vi "Send Set DER Control Msg (Delayed).vi"(7 "Milliseconds To Wait (1000)":i32=1000, 8 "error in":errorcluster, 10 "DER_Control":T1, 11 "SCADA Sub Abstract in":refnum<class "Device Communication and Control Abstract.lvclass">) -> (0 "error out":errorcluster, 3 "dup SCADA Sub Abstract":refnum<class "Device Communication and Control Abstract.lvclass">)   [LabVIEW 2018, in "Device Communication and Control Abstract Actor.lvlib" / "Device Communication and Control Abstract.lvclass"]
uses:
  Device Communication and Control Abstract.lvclass
  C:/Program Files (x86)/National Instruments/LabVIEW 2018/vi.lib/ActorFramework/Actor/Actor.lvclass
  <vilib>/ORNL/CSEISMIC DDS/CSEISMIC DDS Base/Data Types/DER_Control.ctl
  <vilib>/ORNL/CSEISMIC DDS/CSEISMIC DDS Base/Data Types/Controls/DeviceID.ctl
  <vilib>/ActorFramework/Actor/Actor.lvclass/Actor.ctl
  Device Communication and Control Abstract.lvclass/Device Communication and Control Abstract.ctl
  Device Communication and Control Abstract Messages/Set DER Control Msg/Set DER Control Msg.lvclass/Set DER Control Msg.ctl
  Device Communication and Control Abstract Messages/Set DER Control Msg/Set DER Control Msg.lvclass
  C:/Program Files (x86)/National Instruments/LabVIEW 2018/vi.lib/ActorFramework/Message/Message.lvclass
  <vilib>/ActorFramework/Time-Delayed Send Message/Time-Delayed Send Message.vi
  <vilib>/ActorFramework/Actor/Actor.lvclass
  <vilib>/ORNL/CSEISMIC DDS/CSEISMIC DDS Base/CSEISMIC DDS.lvclass
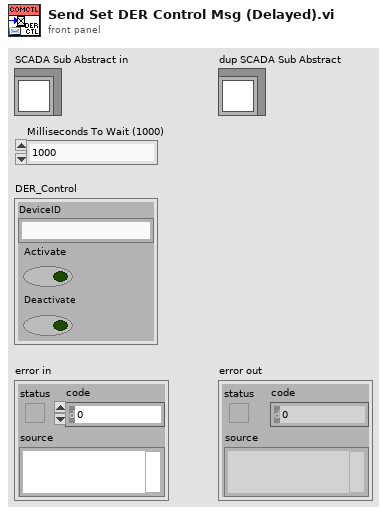
[diagram p1: front panel]
types:
  T1 = typedef "CSEISMIC DDS.lvlib/CSEISMIC DDS.lvclass/DER_Control.ctl" = cluster{"DeviceID":T2, "Activate":bool, "Deactivate":bool}
  T2 = typedef "CSEISMIC DDS.lvlib/CSEISMIC DDS.lvclass/DeviceID.ctl" = string
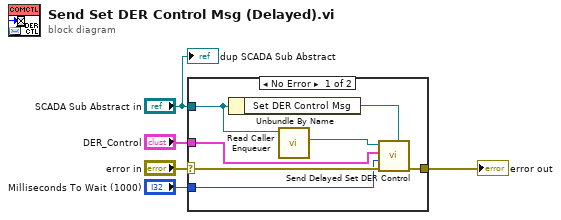
[diagram p0: block diagram]
diagram:
  n1 = case shown="No Error" "error in" {
    selector: "error in" -> [w11 w13]
    tunnel: "SCADA Sub Abstract in" -> [w12 _]
    tunnel: [w10 w13] -> w3
    tunnel: "DER_Control" -> [w7 _]
    tunnel: "Milliseconds To Wait (1000)" -> [w6 _]
    frame No Error {
      n2 = Unbundle By Name(w12) -> ("Set DER Control Msg"=w9:refnum<class "Set DER Control Msg.lvclass">)
      n3 = call <vilib>:"Read Caller Enqueuer.vi"("Actor"=w12) -> ("Caller Enqueuer"=w8:refnum<class "Message Enqueuer.lvclass">)  [unwired: 10 in]
      n4 = call "Send Delayed Set DER Control.vi"("Message Type"=w9, "error in (no error)"=w11, "Milliseconds To Wait"=w6, "DER_Control"=w7, "Message Enqueuer"=w8) -> ("error out"=w10:errorcluster)  [unwired: 5 in, 1 out]
    }
    frame Error {
    }
  }
  "error out" <- w3
  "dup SCADA Sub Abstract" <- "SCADA Sub Abstract in"
